vi "Log Viewer.vi"() -> ()   [LabVIEW 2012]
uses:
  Logging VIs/Equals VIs/Logging Equals - Entries.vi
  femtoRoboLib.lvlib
panel:
  out "Log Path":path
  out "Size (kb)":dbl
  in  "Host":string
  in  "Remote":bool
  in  "Speed":dbl=2.0 min=0.0 step=0.25
  in  "Play":bool
  out "Current":dbl
  out "End":dbl
  in  "Logs":i32(listbox)
  in  "path":path=path "e:/tmp/logs"
  out "Tree":string(tree)
  in  "Time Scrollbar":u32(c297)
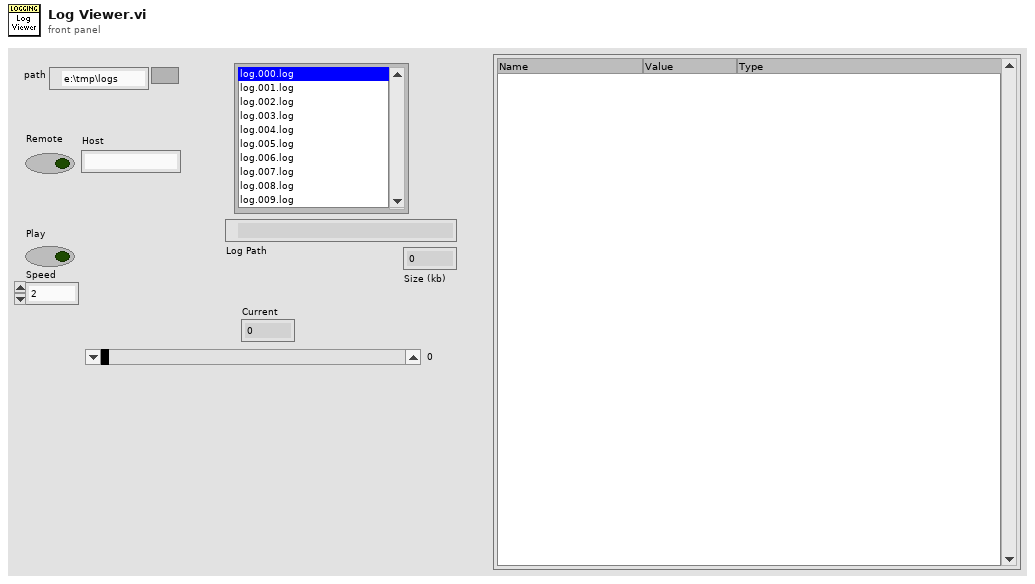
[diagram p1: front panel]
types:
  T1 = typedef "femtoRoboLib.lvlib/LoggingDevRef.ctl" = cluster{"DevStatus":errorcluster, "refnum":refnum<file>, "Path":path, "Start Time":u32}
  T2 = typedef "femtoRoboLib.lvlib/Log Entry - Full Block.ctl" = cluster{"Entries":T3[], "Time":u32}
  T3 = typedef "femtoRoboLib.lvlib/Log Entry.ctl" = cluster{"Name":string, "Type":T4, "Value":T5}
  T4 = typedef "femtoRoboLib.lvlib/Log Value Type.ctl" = enum16{"Boolean", "Numeric", "String", "Boolean Array", "Numeric Array", "String Array"}
  T5 = typedef "femtoRoboLib.lvlib/Log Value Cluster.ctl" = cluster{"Boolean Array":bool[], "Boolean":bool, "Numeric Array":dbl[], "Numeric":dbl, "String Array":string[], "String":string}
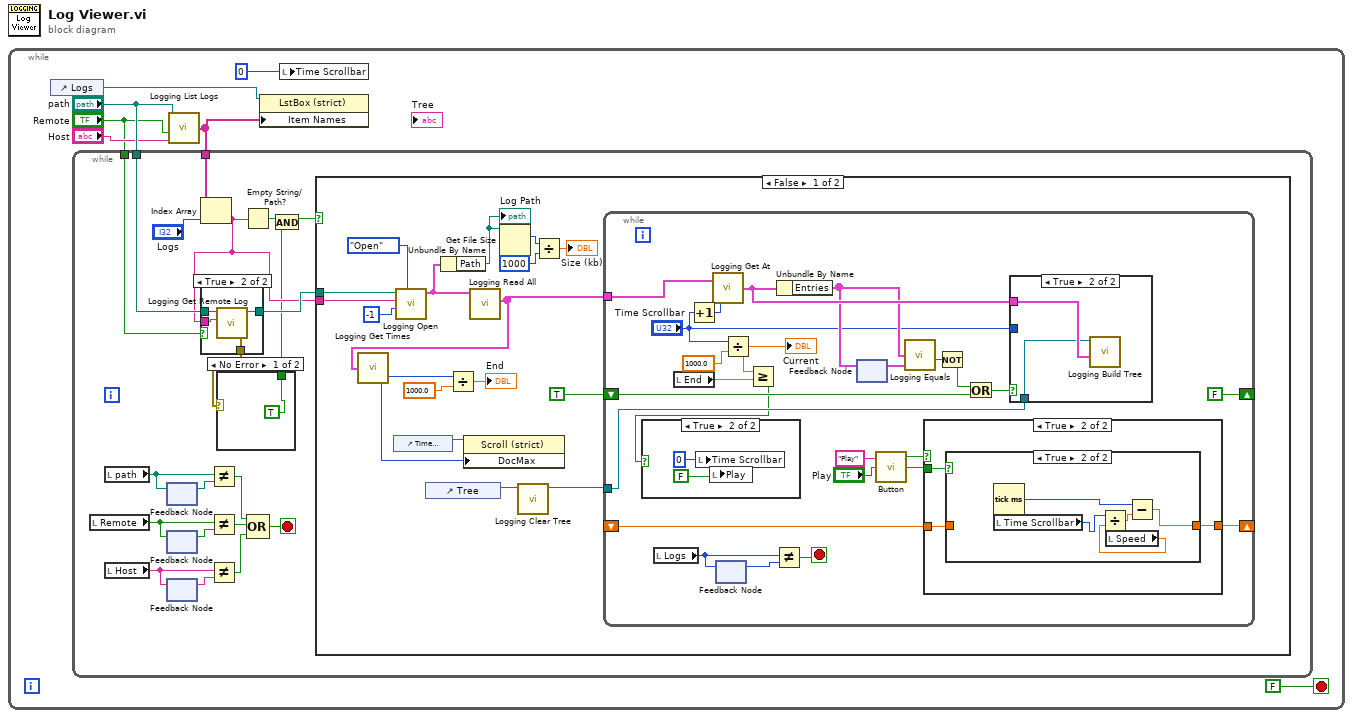
[diagram p0: block diagram]
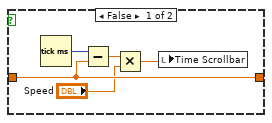
[diagram p6: hidden frame]
diagram:
  n1 = while {
    stop <- FALSE stop-if-true
    n2 = control-ref of="Logs"() -> (w7:refnum<vi>)
    n3 = call "Logging List Logs.vi"("Path"="path", "Remote"="Remote", "Host"="Host") -> ("filenames"=w6:string[])  [unwired: 2 in]
    n4 = while {
      tunnel: w6 -> [w27]
      tunnel: "path" -> [w22]
      tunnel: "Remote" -> [w24]
      stop <- w11 stop-if-true
      n5 = local read "Remote"() -> (w17:bool)
      n6 = local read "path"() -> (w19:path)
      n7 = local read "Host"() -> (w15:string)
      n8 = feedback-in #1(w19) -> ()
      n9 = feedback #1() -> (w20:path)  [unwired: 1 in]
      n10 = feedback #2() -> (w18:bool)  [unwired: 1 in]
      n11 = feedback-in #2(w17) -> ()
      n12 = feedback #3() -> (w16:string)  [unwired: 1 in]
      n13 = feedback-in #3(w15) -> ()
      n14 = Index Array(array=w27, index="Logs") -> (element=w21:string)
      n15 = case shown="True" w24 {
        tunnel: [w29 w33] -> w23
        tunnel: w22 -> [w29 w32]
        tunnel: w21 -> [_ w31]
        tunnel: [_ w30] -> w10
        frame False {
        }
        frame True {
          n16 = call "Logging Get Remote Log.vi"("Name"=w31, "Path"=w32) -> ("error out"=w30:errorcluster, "Path out"=w33:path)  [unwired: 3 in, 1 out]
        }
      }
      n17 = Not Equal?(x=w19, y=w20) -> (x != y?=w14:bool)
      n18 = Not Equal?(x=w17, y=w18) -> (x != y?=w13:bool)
      n19 = Not Equal?(x=w15, y=w16) -> (x != y?=w12:bool)
      n20 = case shown="No Error" w10 {
        tunnel: [TRUE _] -> w8
        frame No Error {
        }
        frame Error {
        }
      }
      n21 = Empty String/Path?(string/path=w21) -> (empty?=w25:bool)
      n22 = Compound Arithmetic op=OR(w14, w13, w12) -> (w11:bool)
      n23 = And(x=w25, y=w8) -> (x .and. y?=w9:bool)
      n24 = case shown="False" w9 {
        tunnel: w23 -> [w40 _]
        tunnel: w21 -> [w41 _]
        frame False {
          n25 = control-ref of="Time Scrollbar"() -> (w47:refnum<vi>)
          n26 = call "Logging Open.vi"("Mode"=enum16{"Create", "Open"}."Open", "Number"=-1, "name"=w41, "base path"=w40) -> ("LoggingDevRef"=w35:T1)  [unwired: 5 in, 1 out]
          n27 = control-ref of="Tree"() -> (w50:refnum<vi>)
          n28 = Unbundle By Name(w35) -> ("Path"=w34:path)
          "Log Path" <- w34
          n29 = call "Logging Read All.vi"("LoggingDevRef"=w35) -> ("Log"=w48:T2[])  [unwired: 4 in, 2 out]
          n30 = call "Logging Get Times.vi"("Log Input"=w48) -> ("Latest"=w44:u32)  [unwired: 1 out]
          n31 = Divide(x=w44, y=1000.0) -> (x/y=→"End":dbl)
          n32 = property class="Scroll (strict)"(reference=w47, "DocMax"=w44) -> ()  [unwired: 1 in, 2 out]
          n33 = Get File Size(file=w34) -> (size (in bytes)=w39:i64)  [unwired: 1 in, 2 out]
          n34 = call "Logging Clear Tree.vi"("TreeRef"=w50) -> ("TreeRef"=w49:refnum<vi>)  [unwired: 6 in]
          n35 = Divide(x=w39, y=i64 1000) -> (x/y=→"Size (kb)":dbl)
          n36 = while {
            tunnel: w48 -> [w73]
            tunnel: w49 -> [w75]
            shift-right: [FALSE] -> _
            shift-left: TRUE -> [w64]
            shift-right: [w59] -> _
            shift-left: _ -> [w58]
            stop <- w67 stop-if-true
            n37 = local read "Logs"() -> (w69:i32)
            n38 = local read "End"() -> (w52:dbl)
            n39 = Increment(x="Time Scrollbar") -> (x+1=w56:u32)
            n40 = call "Logging Get At.vi"("Time (ms)"=w56, "Log Input"=w73) -> ("Output"=w71:T2)
            n41 = feedback-in #4(w69) -> ()
            n42 = feedback #4() -> (w68:i32)  [unwired: 1 in]
            n43 = Divide(x="Time Scrollbar", y=1000.0) -> (x/y=w53:dbl)
            "Current" <- w53
            n44 = Greater Or Equal?(x=w53, y=w52) -> (x >= y?=w51:bool)
            n45 = case shown="True" w51 {
              frame False {
              }
              frame True {
                n46 = local write "Time Scrollbar"(u32 0 ("Time Scrollbar")) -> ()
                n47 = local write "Play"(FALSE) -> ()
              }
            }
            n48 = Not Equal?(x=w69, y=w68) -> (x != y?=w67:bool)
            n49 = Unbundle By Name(w71) -> ("Entries"=w70:T3[])
            n50 = feedback-in #5(w70) -> ()
            n51 = feedback #5() -> (w72:T3[])  [unwired: 1 in]
            n52 = call "Button.vi"("In"="Play", "Name"="Play") -> ("Leading"=w60:bool, "Out"=w61:bool)  [unwired: 1 in, 1 out]
            n53 = call-poly "Logging Equals.vi"("Entries A"=w70, "Entries B"=w72) -> ("Equal"=w66:bool)  [unwired: 4 in]
            n54 = case shown="True" w61 {
              tunnel: w60 -> [_ w80]
              tunnel: [_ w79] -> w59
              tunnel: w58 -> [_ w78]
              frame False {
              }
              frame True {
                n55 = case shown="True" w80 {
                  tunnel: [w84 w89] -> w79
                  tunnel: w78 -> [w84 _]
                  frame False {
                    n56 = Tick Count (ms)() -> (millisecond timer value=w85:u32)
                    n57 = Subtract(x=w85, y=w84) -> (x-y=w83:dbl)
                    n58 = Multiply(x=w83, y="Speed") -> (x*y=w81:dbl)
                    n59 = local write "Time Scrollbar"(w81) -> ()
                  }
                  frame True {
                    n60 = Tick Count (ms)() -> (millisecond timer value=w90:u32)
                    n61 = local read "Time Scrollbar"() -> (w86:u32)
                    n62 = local read "Speed"() -> (w87:dbl)
                    n63 = Divide(x=w86, y=w87) -> (x/y=w88:dbl)
                    n64 = Subtract(x=w90, y=w88) -> (x-y=w89:dbl)
                  }
                }
              }
            }
            n65 = Not(x=w66) -> (.not. x?=w63:bool)
            n66 = Or(x=w63, y=w64) -> (x .or. y?=w65:bool)
            n67 = case shown="True" w65 {
              tunnel: w75 -> [_ w91]
              tunnel: "Time Scrollbar" -> [_ _]
              tunnel: w71 -> [_ w92]
              frame False {
              }
              frame True {
                n68 = call "Logging Build Tree.vi"("Entries"=w92, "TreeRef"=w91) -> ()  [unwired: 5 in, 1 out]
              }
            }
          }
        }
        frame True {
        }
      }
    }
    n69 = property class="LstBox (strict)"(reference=w7, "Item Names"=w6) -> ()  [unwired: 1 in, 2 out]
    n70 = local write "Time Scrollbar"(0) -> ()
  }
